vi "Configure Ethernet.vi"(8 "error in (no error)":errorcluster, 9 "Ethernet configuration":T1, 10 "hardware interface index":u16, 11 "PLBB in":refnum<class "PL BlackBox Modbus Client.lvclass">) -> (0 "error out":errorcluster, 3 "PLBB out":refnum<class "PL BlackBox Modbus Client.lvclass">)   [LabVIEW 2015, in "PL BlackBox Modbus Client.lvclass"]
doc: "Configures the Ethernet."
uses:
  PL BlackBox Modbus Client.lvclass
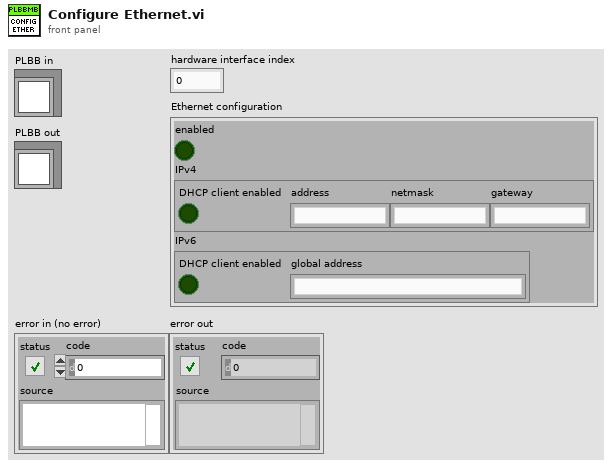
[diagram p1: front panel]
types:
  T1 = cluster{"enabled":bool, "IPv4":cluster{"DHCP client enabled":bool, "address":string, "netmask":string, "gateway":string}, "IPv6":cluster{"DHCP client enabled":bool, "global address":string}}
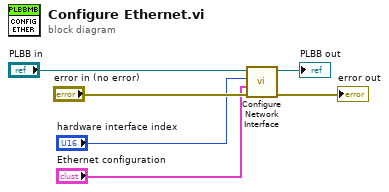
[diagram p0: block diagram]
diagram:
  n1 = call "Configure Network Interface.vi"("error in (no error)"="error in (no error)", "network interface configuration"="Ethernet configuration", "hardware interface index"="hardware interface index", "PLBB in"="PLBB in") -> ("error out"=→"error out":errorcluster, "PLBB out"=→"PLBB out":refnum<class "PL BlackBox Modbus Client.lvclass">)  [unwired: 6 in]
